vi "Create and Fire Initialization Event.vi"() -> (3 "Event Registration Refnum out":refnum<event-registration>)   [LabVIEW 2014]
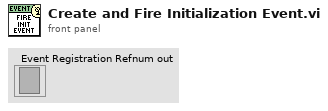
[diagram p1: front panel]
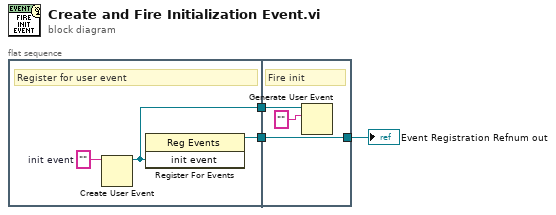
[diagram p0: block diagram]
diagram:
  n1 = flat-sequence {
    tunnel: [w5] -> w3
    tunnel: [w4] -> w2
    tunnel: [w9] -> w1
    tunnel: w3 -> [w9]
    tunnel: w2 -> [w8]
    frame #0 {
      w6 = ""  # init event
      # "Register for user event"
      n2 = Create User Event(user event datatype=w6) -> (user event=w4:refnum<user-event>)  [unwired: 1 in, 1 out]
      n3 = register-events(w4) -> (reference out=w5:refnum<event-registration>)  [unwired: 2 in, 1 out]
    }
    frame #1 {
      # "Fire init"
      n4 = Generate User Event(user event=w8, event data cluster="" ("event data")) -> ()  [unwired: 2 in, 2 out]
    }
  }
  "Event Registration Refnum out" <- w1
